vi "rejectedCommandEvent.vi"(8 "error in (no error)":errorcluster, 9 "State in":refnum<class "ElectrometerState.lvclass">, 10 "InternalCommandId.lvclass":refnum<class "InternalCommandId.lvclass">, 11 "ElectrometerController in":refnum<class "ElectrometerController.lvclass">) -> (0 "error out":errorcluster, 3 "ElectrometerController out":refnum<class "ElectrometerController.lvclass">)   [LabVIEW 2016, in "ElectrometerController.lvclass"]
uses:
  ElectrometerController.lvclass
  InternalCommandId/InternalCommandId.lvclass
  Electrometer/State/ElectrometerState.lvclass
  ts_sallv_calibrationelectrometer/DataTypes/logevent_rejectedCommand.ctl
  ElectrometerController.lvclass/ElectrometerController.ctl
  ts_sallv_calibrationelectrometer/SALLV_calibrationElectrometer.lvlib
  ts_electrometeruserevents/MiddlewareSALThisComponent/MiddlewareSALThisComponent.lvclass
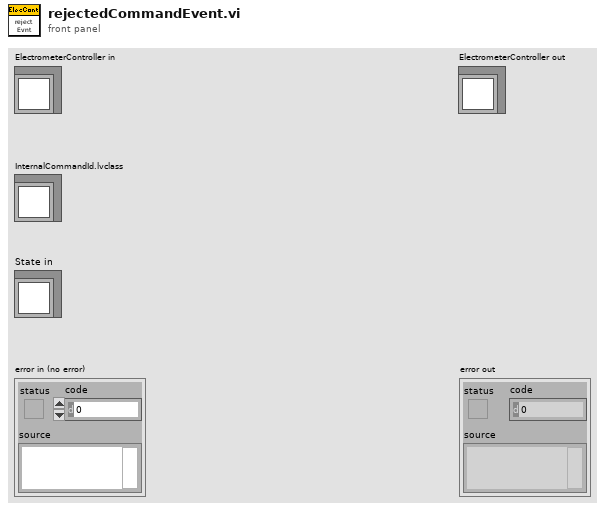
[diagram p1: front panel]
types:
  T1 = typedef "SALLV_calibrationElectrometer.lvlib/logevent_rejectedCommand.ctl" = cluster{"commandValue":u16, "detailedState":u16, "timestamp":dbl, "electId":string, "priority":i32}
  T2 = typedef "ElectrometerTypedefs.lvlib/StateValue.ctl" = enum16{"", "DisabledState", "EnabledState", "FaultState", "OffState", "StandbyState", "ReadyState", "ConfiguringState", "ManualReadingState", "UntilIntensityReadingState", "SetDurationReadingState", "BufferReadingState"}
  T3 = typedef "ElectrometerTypedefs.lvlib/CommandValue.ctl" = enum16{"N/A", "Disable", "Enable", "Exit", "GoToStandby", "OnHeartbeat", "OnIncomingMessagingError", "OnInterrupt", "Start", "SetDigitalFilter", "StartScan", "StartScanDt", "StartScanReachIntensity", "StopScan", "SetIntegrationTime", "PerformZeroCalib", "SetRange", "SetMode", "Power"}
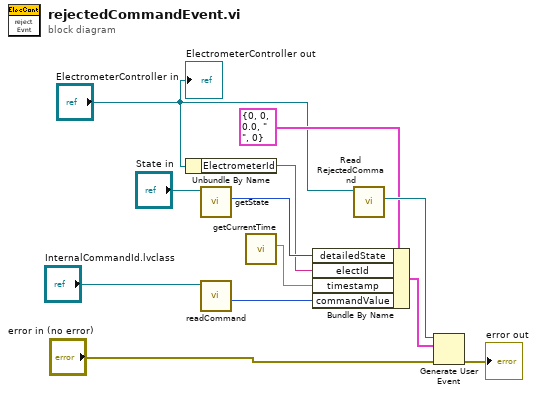
[diagram p0: block diagram]
diagram:
  n1 = Unbundle By Name("ElectrometerController in") -> ("ElectrometerId"=w2:string)
  n2 = call-dynamic "getState.vi"("State in"="State in") -> ("StateValue"=w4:T2)  [unwired: 8 in, 2 out]
  n3 = call "readCommand.vi"("InternalCommandId in"="InternalCommandId.lvclass") -> ("CommandValue"=w5:T3)  [unwired: 7 in, 3 out]
  n4 = call "getCurrentTime.vi"() -> ("timestamp"=w1:dbl)  [unwired: 9 in, 2 out]
  n5 = Bundle By Name(cluster=T1 {"commandValue"=0, "detailedState"=0, "timestamp"=0.0, "electId"="                                                                                                                                                                                                                                                                ", "priority"=0} ("event data"), "detailedState"=w4, "electId"=w2, "timestamp"=w1, "commandValue"=w5) -> (w7:T1)
  n6 = call-dynamic "Read RejectedCommand.vi"("ElectrometerController in"="ElectrometerController in") -> ("RejectedCommand"=w10:refnum<user-event>)  [unwired: 8 in, 2 out]
  n7 = Generate User Event(user event=w10, event data cluster=w7, error in="error in (no error)") -> (error out=→"error out":errorcluster)  [unwired: 1 in, 1 out]
  "ElectrometerController out" <- "ElectrometerController in"
